vi "Error Write Watch.vi"(8 "error in":errorcluster, 10 "Watchdog STS":i32, 11 "Power Supply In":refnum<class "Power Supply.lvclass">) -> (0 "error out":errorcluster, 3 "Power Supply Out":refnum<class "Power Supply.lvclass">)   [LabVIEW 2023, in "Power Supply.lvclass"]
uses:
  Power Supply.lvclass
  Power Supply.lvclass/Power Supply.ctl
  Low Level Capabilities/Error/Error.lvclass
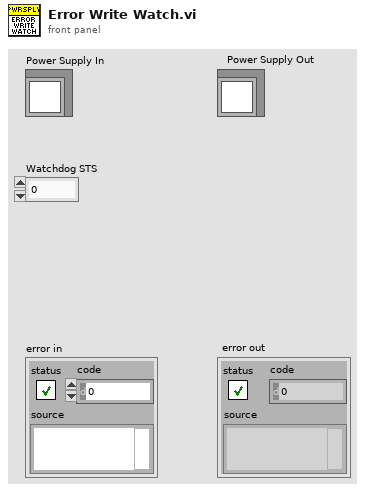
[diagram p1: front panel]
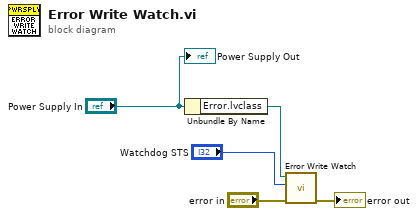
[diagram p0: block diagram]
diagram:
  n1 = Unbundle By Name("Power Supply In") -> ("Error.lvclass"=w1:refnum<class "Error.lvclass">)
  n2 = call-dynamic "Error Write Watch.vi"("error in"="error in", "Watchdog STS"="Watchdog STS", "Error in"=w1) -> ("error out"=→"error out":errorcluster)  [unwired: 7 in, 1 out]
  "Power Supply Out" <- "Power Supply In"
